vi "Handle Command.vi"(8 "error in":errorcluster, 10 "CMD in":refnum<class "Update Serialize Waverform CMD.lvclass">, 11 "Object In":refnum<class>) -> (0 "error out":errorcluster, 1 "Command Successful?":bool, 2 "CMD out":refnum<class "Update Serialize Waverform CMD.lvclass">, 3 "Object Out":refnum<class>)   [LabVIEW 2017, in "gPAS Library.lvlib" / "Update Serialize Waverform CMD.lvclass"]
doc: "This VI will contain the code used to actually execute the request. If the request is successful, this will be indicated by the boolean output <b>Command Successful?</b>. The boolean output can then be used by the <b>Command Reply</b> which sends a reply if the reply queue is valid."
uses:
  Update Serialize Waverform CMD.lvclass
  <vilib>/MSR Consulting, LLC/General Reuse/PAS/Main/PAS.lvclass
  C:/Program Files (x86)/National Instruments/LabVIEW 2017/vi.lib/MSR Consulting, LLC/General Reuse/Instrument/Instrument.lvclass
  <vilib>/MSR Consulting, LLC/General Reuse/PAS/Data/Main/PAS Data.lvclass
  C:/Program Files (x86)/National Instruments/LabVIEW 2017/vi.lib/MSR Consulting, LLC/General Reuse/Data/Data.lvclass
  Update Serialize Waverform CMD.lvclass/Update Serialize Waverform CMD.ctl
  <vilib>/MSR Consulting, LLC/General Reuse/Instrument/Instrument.lvclass/Instrument.ctl
  <vilib>/MSR Consulting, LLC/General Reuse/PAS/Data/Cell/PAS Cell Data.lvclass/PAS Cell Data.ctl
  <vilib>/MSR Consulting, LLC/General Reuse/PAS/Data/Cell/Write serializeWF_.vi
  <vilib>/MSR Consulting, LLC/General Reuse/Instrument/Write Data.vi
  <vilib>/MSR Consulting, LLC/General Reuse/Instrument/Read Data.vi
  <vilib>/MSR Consulting, LLC/General Reuse/PAS/Data/Main/Read CellData.vi
  <vilib>/MSR Consulting, LLC/General Reuse/PAS/Data/Main/Write CellData.vi
  <vilib>/MSR Consulting, LLC/General Reuse/Data/Data.lvclass
  <vilib>/MSR Consulting, LLC/General Reuse/PAS/Data/Cell/PAS Cell Data.lvclass
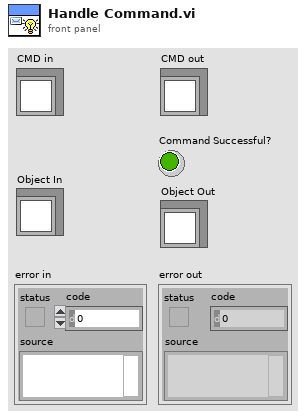
[diagram p1: front panel]
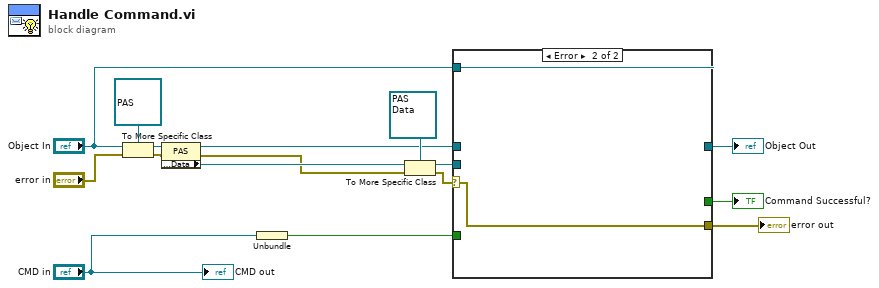
[diagram p0: block diagram]
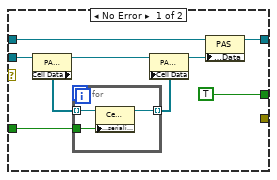
[diagram p2: hidden frame]
diagram:
  n1 = To More Specific Class(target class=refnum<class "PAS.lvclass"> refnum ("PAS Library.lvlib:PAS"), reference="Object In", error in="error in") -> (specific class reference=w15:refnum<class "PAS.lvclass">, error out=w6:errorcluster)
  n2 = property class="PAS"(reference=w15, error in=w6) -> (reference out=w11:refnum<class "PAS.lvclass">, error out=w5:errorcluster, "Accessors:Data"=w13:refnum<class "Data.lvclass">)
  n3 = Unbundle("CMD in") -> (w8:bool)
  n4 = To More Specific Class(target class=refnum<class "PAS Data.lvclass"> refnum ("PAS Library.lvlib:PAS Data"), reference=w13, error in=w5) -> (specific class reference=w12:refnum<class "PAS Data.lvclass">, error out=w4:errorcluster)
  n5 = case shown="Error" w4 {
    selector: w4 -> [_ w29]
    tunnel: w12 -> [w24 _]
    tunnel: w11 -> [w22 _]
    tunnel: [w21 w30] -> w10
    tunnel: w8 -> [w19 _]
    tunnel: "Object In" -> [_ w30]
    tunnel: [TRUE ("Command Successful?") _] -> w2
    tunnel: [_ w29] -> w1
    frame No Error {
      n6 = property class="PAS Data"(reference=w24) -> (reference out=w17:refnum<class "PAS Data.lvclass">, "Cell Data"=w25:refnum<class "PAS Cell Data.lvclass">[])  [unwired: 1 in, 1 out]
      n7 = for {
        tunnel: w25 -> [w28] mode=indexing
        tunnel: [w27] -> w23 mode=indexing
        tunnel: w19 -> [w26]
        n8 = property class="Cell Data"(reference=w28, "Accessors:serializeWF_"=w26) -> (reference out=w27:refnum<class "PAS Cell Data.lvclass">)  [unwired: 1 in, 1 out]
      }
      n9 = property class="PAS Data"(reference=w17, "Cell Data"=w23) -> (reference out=w20:refnum<class "PAS Data.lvclass">)  [unwired: 1 in, 1 out]
      n10 = property class="PAS"(reference=w22, "Accessors:Data"=w20) -> (reference out=w21:refnum<class "PAS.lvclass">)  [unwired: 1 in, 1 out]
    }
    frame Error {
    }
  }
  "error out" <- w1
  "Object Out" <- w10
  "Command Successful?" <- w2
  "CMD out" <- "CMD in"
